vi "Custom Trigger AI.vi"() -> ()   [LabVIEW 2010]
uses:
  <vilib>/eio/EIONode/EIONode.xnode
  <vilib>/rvi/eio/nirviEIOImplementation/nirviEIOImplementation.xnode
  <vilib>/rvi/eio/common/nirviEmuClasses.ctl
  <vilib>/rvi/DataTransferAndStorage/Container/XNode/niFpgaContainer.xnode
  <vilib>/rvi/DataTransferAndStorage/Container/Common/niFpgaContainerMethod.ctl
  <vilib>/rvi/DataTransferAndStorage/Container/Common/niFpgaTransferTypeControl.ctl
  <vilib>/rvi/eio/common/nirviEmuTemplateMethod_noerrors.vi
  <vilib>/rvi/interface/RandomDataEmulation/nirviRandomDataFPGAFIFO.vi
  <vilib>/rvi/interface/RandomDataEmulation/niFpgaRandomDataHandleErrors.vi
panel:
  in  "Stop":bool
  in  "AI Threshold Low":i16
  in  "Trigger Enable":bool
  out "Overflow\nOccurred?":bool
  in  "Number of Samples":i32
  in  "FPGA Sample Period (us)":u32
  in  "AI Threshold High":i16
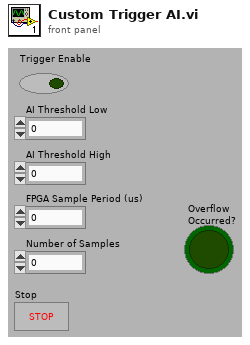
[diagram p1: front panel]
types:
  T1 = typedef "niFpgaContainerMethod.ctl" = enum16{"<none>", "write", "read", "clear", "getNumberOfElementsToWrite", "getNumberOfElementsToRead", "enable", "disable", "flushAndDisable", "getStreamState", "readA", "readB", "dramWrite", "dramWriteWithByteEnables", "dramRequestData", "dramRetrieveData"}
  T2 = typedef "niFpgaTransferTypeControl.ctl" = enum16{"Target-Scoped", "Host to Target - DMA", "Target to Host - DMA", "Peer to Peer Reader", "Peer to Peer Writer", "Bidirectional"}
  T3 = typedef "nirviEmuClasses.ctl" = enum16{"IO Read", "IO Write", "Method", "Property Read", "Property Write"}
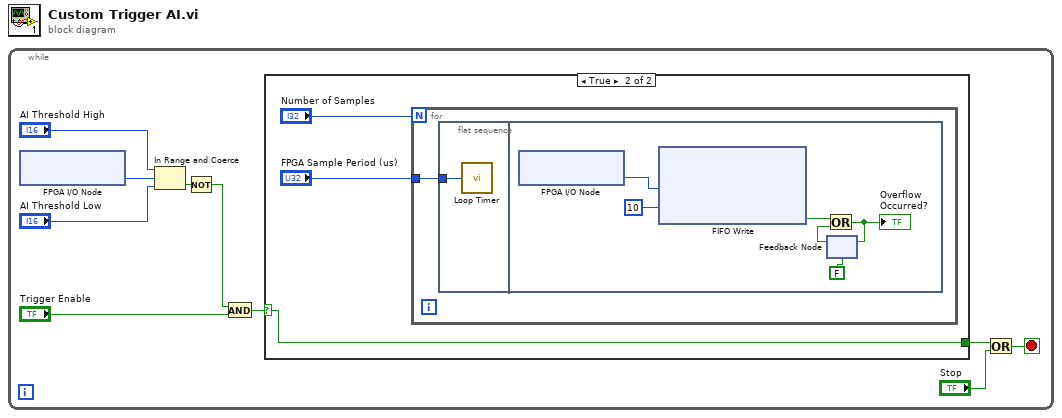
[diagram p0: block diagram]
diagram:
  n1 = while {
    stop <- w3 stop-if-true
    n2 = xnode "FPGA I/O Node"() -> ("Analog Input"=w7:i16)  [unwired: 1 in, 1 out]
    n3 = In Range and Coerce(upper limit="AI Threshold High", x=w7, lower limit="AI Threshold Low") -> (In Range?=w8:bool)  [unwired: 1 out]
    n4 = Not(x=w8) -> (.not. x?=w6:bool)
    n5 = And(x=w6, y="Trigger Enable") -> (x .and. y?=w10:bool)
    n6 = case shown="True" w10 {
      selector: w10 -> [w11 w12]
      tunnel: [w11 w12] -> w2
      frame False {
      }
      frame True {
        n7 = for {
          N: "Number of Samples" -> [_]
          tunnel: "FPGA Sample Period (us)" -> [w15]
          n8 = flat-sequence {
            tunnel: w15 -> [w16]
            frame #0 {
              n9 = call "Loop Timer"("Count(uSec)"=w16) -> ()  [unwired: 1 out]
            }
            frame #1 {
              n10 = xnode "FPGA I/O Node"() -> ("Analog Input"=w22:i16)  [unwired: 1 in, 1 out]
              n11 = xnode ("FIFO Write")("Element"=w22, "Timeout"=10) -> ("Timed Out?"=w20:bool)  [unwired: 1 in, 1 out]
              n12 = feedback #1(FALSE) -> (w19:bool)
              n13 = Or(x=w20, y=w19) -> (x .or. y?=w18:bool)
              "Overflow\nOccurred?" <- w18
              n14 = feedback-in #1(w18) -> ()
            }
          }
        }
      }
    }
    n15 = Or(x=w2, y="Stop") -> (x .or. y?=w3:bool)
  }
